vi "Sweep control.vi"(0 "Scan control":cluster{"Priority":u16, "Scan name":u16}[](array[cluster])=[{"Priority"=0, "Scan name"=1}, {"Priority"=3, "Scan name"=0}, {"Priority"=2, "Scan name"=0}, {"Priority"=1, "Scan name"=5}] {"Scan name" items=["OFF", "Vsg1", "Vsg2", "Vsgw", "Vbg", "Field", "Temp"]; "Priority" items=["Priority 0", "Priority 1", "Priority 2", "Priority 3", "Priority 4", "Priority 5"]}, 1 "Scan parameters":T2(array[cluster])=[{"DAQ Channel"=1, "Label"="\nappliedVsg=", "Scaled low"=-0.1, "Scaled high"=0.1, "Start"=0.0, "End"=0.18, "Step"=0.0001, "Scale?"=FALSE}, {"DAQ Channel"=2, "Label"="\nappliedTemperature=", "Scaled low"=-0.175, "Scaled high"=0.775, "Start"=0.1, "End"=0.9, "Step"=0.1, "Scale?"=FALSE}, {"DAQ Channel"=3, "Label"="\nappliedVbg=", "Scaled low"=-0.11, "Scaled high"=0.31, "Start"=-0.5, "End"=0.5, "Step"=0.001, "Scale?"=FALSE}, {"DAQ Channel"=3, "Label"="\nappliedField=", "Scaled low"=-0.060000000000000005, "Scaled high"=0.14, "Start"=-10000.0, "End"=0.0, "Step"=2000.0, "Scale?"=FALSE}] {"Step" format="%#_6f"; "End" format="%#_6f"; "Start" format="%#_6f"; "Scaled high" format="%#_6p"; "Scaled low" format="%#_6p"}, 2 "OSC Configuration":T1(array[cluster])=[{"Signal Type"=enum."Sawtooth Wave", "DC"=0.00034, "Amplitude"=0.0015, "frequency"=0.4, "Phase"=180.0}, {"Signal Type"=enum."Sine Wave", "DC"=0.0, "Amplitude"=0.0, "frequency"=1.0, "Phase"=0.0}, {"Signal Type"=enum."Sine Wave", "DC"=0.0, "Amplitude"=0.0, "frequency"=1.0, "Phase"=0.0}, {"Signal Type"=enum."Sine Wave", "DC"=0.0, "Amplitude"=0.0, "frequency"=1.0, "Phase"=0.0}] {"frequency" format="%0.2p"; "Amplitude" format="%0.2p"; "DC" format="%.2p"}, 3 "Comments":string="SA02704G.20140716\nbackgate=0V", 4 "Experiment folder name":string="3- sweep Vsg_50mK_field", 8 "Additional action (indexing priority)":u16[](array[ring])=[4, 2, 4, 4] items=["Clear DAQ Tasks", "Check Temperature", "Check Field Value", "Wait", "Do Nothing"]) -> ()   [LabVIEW 2013]
uses:
  <userlib>/LevyLab/PPMS_VIs/Lockin-4461_MultiChannel - IV 3.0 globals.vi
panel:
  in  "Number of IV curves":i32=1
  # "Instructions: \n1, you can put multiple scan names in one priority.\n2 OFF has to put in last priority"
  # "I wanted to check the temperature as well as the field (so the zero-field data isn't taken at higher temperatures) so I changed the post-action subvi slightly. In the 'check temperature' case, I made the stop condition that the temp is less than 70mK. By putting 'check temperature' with priority 1, i figure it'll set Vsg1&2 at 0, then wait for the temp to reach 70mK, before it starts sweeping prioity 0."
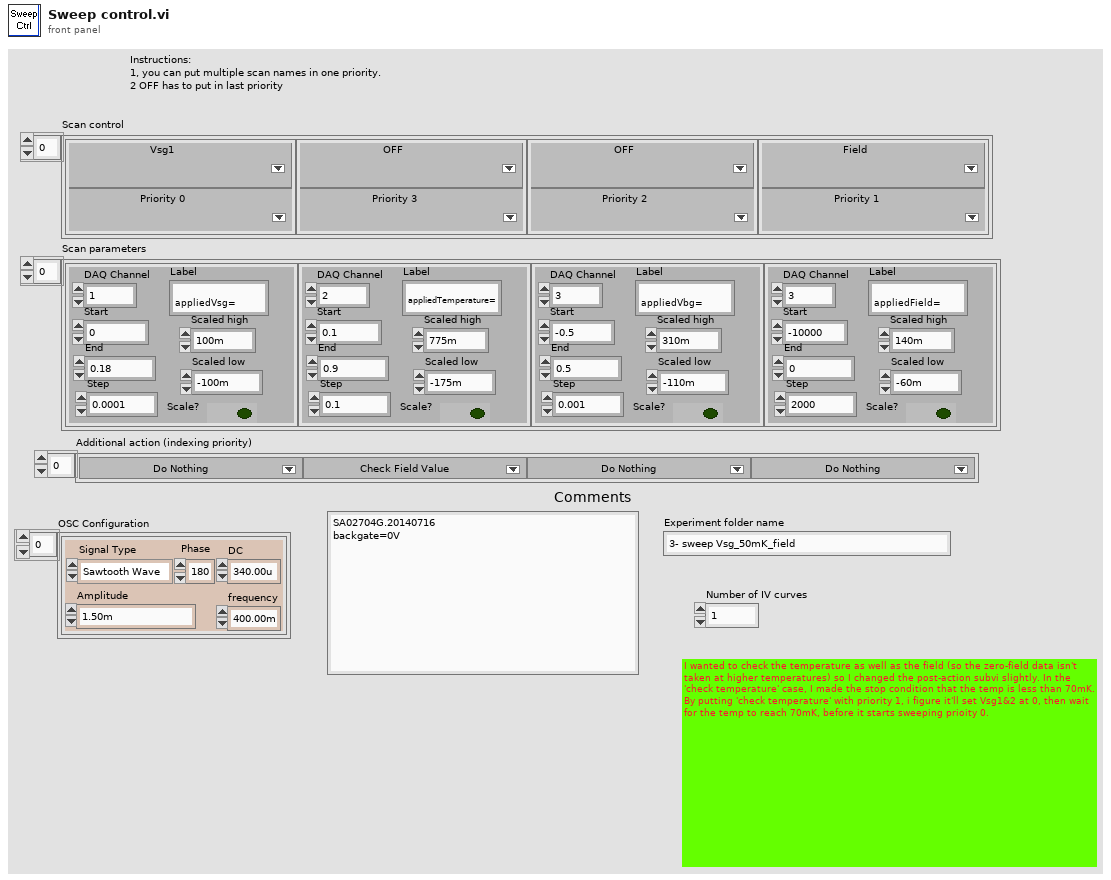
[diagram p1: front panel]
types:
  T1 = cluster{"Signal Type":enum16{"Sine Wave", "Triangle Wave", "Square Wave", "Sawtooth Wave"}, "DC":dbl, "Amplitude":dbl, "frequency":dbl, "Phase":dbl}[]
  T2 = cluster{"DAQ Channel":i32, "Label":string, "Scaled low":dbl, "Scaled high":dbl, "Start":dbl, "End":dbl, "Step":dbl, "Scale?":bool}[]
  T3 = cluster{cluster{"DAQ Channel":i32, "Label":string, "Scaled low":dbl, "Scaled high":dbl, "Start":dbl, "End":dbl, "Step":dbl, "Scale?":bool}[]}[]
  T4 = cluster{cluster{"Priority":u16, "Scan name":u16}[]}[]
  T5 = cluster{cluster{"DAQ Channel":i32, "Label":string, "Scaled low":dbl, "Scaled high":dbl, "Start":dbl, "End":dbl, "Step":dbl, "Scale?":bool}[]}
  T6 = cluster{cluster{"Priority":u16, "Scan name":u16}[]}
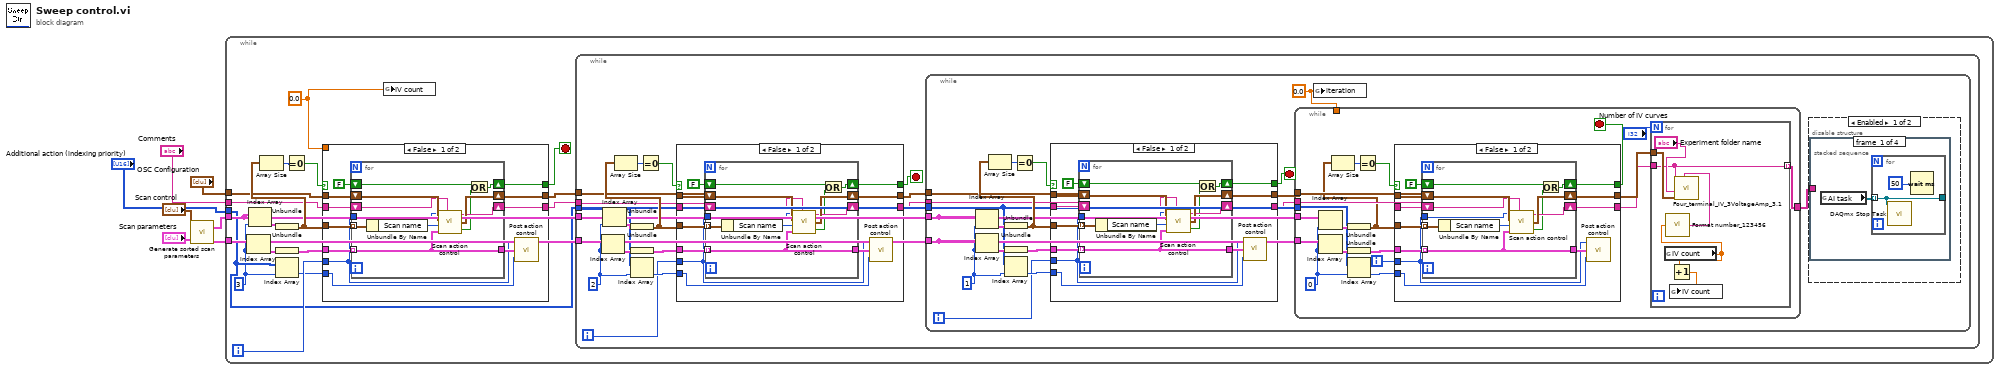
[diagram p0: block diagram]
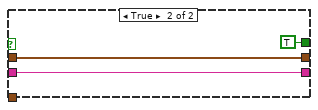
[diagram p2: hidden frame]
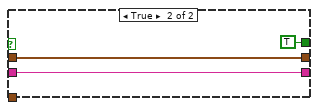
[diagram p3: hidden frame]
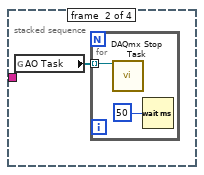
[diagram p4: hidden frame]
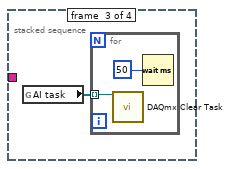
[diagram p5: hidden frame]
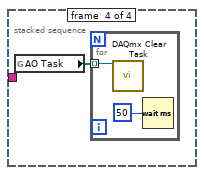
[diagram p6: hidden frame]
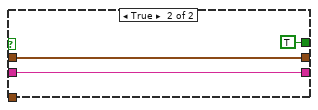
[diagram p8: hidden frame]
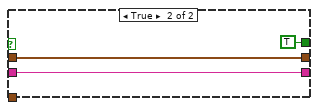
[diagram p9: hidden frame]
diagram:
  n1 = call "Generate sorted scan parameters.vi"("Scan parameters"="Scan parameters", "Scan control"="Scan control") -> ("Sorted scan parameters"=w3:T3, "Sorted scan control"=w2:T4)
  n2 = while {
    tunnel: "Comments" -> [w12]
    tunnel: "OSC Configuration" -> [w13]
    tunnel: w3 -> [w20]
    tunnel: w2 -> [w19]
    tunnel: "Additional action (indexing priority)" -> [w14]
    i -> [w16]
    stop <- w17 stop-if-true
    w8 = 0.0 ("IV count")
    w9 = 3
    n3 = Index Array(array=w20, index=w9) -> (element=w21:T5)
    n4 = Index Array(array=w19, index=w9) -> (element=w18:T6)
    n5 = Unbundle(w18) -> (w23:cluster{"Priority":u16, "Scan name":u16}[])
    n6 = Array Size(array=w23) -> (size(s)=w24:i32)
    n7 = Unbundle(w21) -> (w22:T2)
    n8 = Index Array(array=w14, index=w9) -> (element=w15:u16)
    n9 = Equal To 0?(x=w24) -> (x = 0?=w25:bool)
    n10 = case shown="False" w25 {
      tunnel: w22 -> [w36 _]
      tunnel: [w35 w49] -> w11
      tunnel: [w34 w48] -> w10
      tunnel: [w28 TRUE ("Stop?")] -> w17
      tunnel: w23 -> [w33 _]
      tunnel: w16 -> [w30 _]
      tunnel: w15 -> [w31 _]
      tunnel: w13 -> [w27 w49]
      tunnel: w12 -> [w26 w48]
      tunnel: w8 -> [_ _]
      frame False {
        n11 = for {
          tunnel: w33 -> [w47] mode=indexing
          tunnel: w36 -> [w40] mode=indexing
          tunnel: w30 -> [w41]
          shift-right: [w45] -> w35
          shift-left: w27 -> [w44]
          shift-right: [w43] -> w34
          shift-left: w26 -> [w42]
          tunnel: [w40] -> w32
          shift-right: [w37] -> w28
          shift-left: FALSE -> [w39]
          n12 = Unbundle By Name(w47) -> ("Scan name"=w46:u16)
          n13 = call "Scan action control.vi"("Index"=w41, "OSC Configuration"=w44, "Scan control"=w46, "Scan Parameters"=w40, "Comments"=w42) -> ("Comments out"=w43:string, "OSC Configuration out"=w45:T1, "Stop?"=w38:bool)
          n14 = Or(x=w39, y=w38) -> (x .or. y?=w37:bool)
        }
        n15 = call "Post action control.vi"("Action"=w31, "Scan Parameters"=w32, "Index"=w30) -> ()  [unwired: 1 out]
      }
      frame True {
      }
    }
    n16 = global write "Lockin-4461_MultiChannel - IV 3.0 globals.vi" "IV count"(w8) -> ()
    n17 = while {
      tunnel: w20 -> [w60]
      tunnel: w19 -> [w59]
      tunnel: w14 -> [w58]
      tunnel: w10 -> [w57]
      tunnel: w11 -> [w56]
      i -> [w55]
      stop <- w54 stop-if-true
      w51 = 2
      n18 = Index Array(array=w60, index=w51) -> (element=w66:T5)
      n19 = Index Array(array=w59, index=w51) -> (element=w67:T6)
      n20 = Unbundle(w67) -> (w64:cluster{"Priority":u16, "Scan name":u16}[])
      n21 = Array Size(array=w64) -> (size(s)=w62:i32)
      n22 = Unbundle(w66) -> (w65:T2)
      n23 = Index Array(array=w58, index=w51) -> (element=w63:u16)
      n24 = Equal To 0?(x=w62) -> (x = 0?=w61:bool)
      n25 = case shown="False" w61 {
        tunnel: w65 -> [w78 _]
        tunnel: w56 -> [w77 w92]
        tunnel: w57 -> [w76 w91]
        tunnel: [w75 w92] -> w53
        tunnel: [w74 w91] -> w52
        tunnel: [w68 TRUE ("Stop?")] -> w54
        tunnel: w64 -> [w73 _]
        tunnel: w55 -> [w70 _]
        tunnel: w63 -> [w71 _]
        frame False {
          n26 = for {
            tunnel: w73 -> [w89] mode=indexing
            tunnel: w78 -> [w82] mode=indexing
            tunnel: w70 -> [w83]
            shift-right: [w87] -> w75
            shift-left: w77 -> [w86]
            shift-right: [w85] -> w74
            shift-left: w76 -> [w84]
            tunnel: [w82] -> w72
            shift-right: [w79] -> w68
            shift-left: FALSE -> [w81]
            n27 = Unbundle By Name(w89) -> ("Scan name"=w88:u16)
            n28 = call "Scan action control.vi"("Index"=w83, "OSC Configuration"=w86, "Scan control"=w88, "Scan Parameters"=w82, "Comments"=w84) -> ("Comments out"=w85:string, "OSC Configuration out"=w87:T1, "Stop?"=w80:bool)
            n29 = Or(x=w81, y=w80) -> (x .or. y?=w79:bool)
          }
          n30 = call "Post action control.vi"("Action"=w71, "Scan Parameters"=w72, "Index"=w70) -> ()  [unwired: 1 out]
        }
        frame True {
        }
      }
      n31 = while {
        tunnel: w53 -> [w102]
        tunnel: w52 -> [w101]
        tunnel: w59 -> [w100]
        tunnel: w60 -> [w99]
        tunnel: w58 -> [w98]
        i -> [w93]
        stop <- w95 stop-if-true
        w94 = 1
        w111 = 0.0 ("iteration")
        n32 = Index Array(array=w100, index=w94) -> (element=w103:T6)
        n33 = Index Array(array=w99, index=w94) -> (element=w104:T5)
        n34 = Unbundle(w103) -> (w106:cluster{"Priority":u16, "Scan name":u16}[])
        n35 = Array Size(array=w106) -> (size(s)=w108:i32)
        n36 = Unbundle(w104) -> (w105:T2)
        n37 = Index Array(array=w98, index=w94) -> (element=w107:u16)
        n38 = Equal To 0?(x=w108) -> (x = 0?=w109:bool)
        n39 = case shown="False" w109 {
          tunnel: w105 -> [w135 _]
          tunnel: w102 -> [w134 w149]
          tunnel: w101 -> [w133 w148]
          tunnel: [w132 w149] -> w96
          tunnel: [w131 w148] -> w97
          tunnel: [w125 TRUE ("Stop?")] -> w95
          tunnel: w106 -> [w130 _]
          tunnel: w93 -> [w127 _]
          tunnel: w107 -> [w128 _]
          frame False {
            n40 = for {
              tunnel: w130 -> [w146] mode=indexing
              tunnel: w135 -> [w139] mode=indexing
              tunnel: w127 -> [w140]
              shift-right: [w144] -> w132
              shift-left: w134 -> [w143]
              shift-right: [w142] -> w131
              shift-left: w133 -> [w141]
              tunnel: [w139] -> w129
              shift-right: [w136] -> w125
              shift-left: FALSE -> [w138]
              n41 = Unbundle By Name(w146) -> ("Scan name"=w145:u16)
              n42 = call "Scan action control.vi"("Index"=w140, "OSC Configuration"=w143, "Scan control"=w145, "Scan Parameters"=w139, "Comments"=w141) -> ("Comments out"=w142:string, "OSC Configuration out"=w144:T1, "Stop?"=w137:bool)
              n43 = Or(x=w138, y=w137) -> (x .or. y?=w136:bool)
            }
            n44 = call "Post action control.vi"("Action"=w128, "Scan Parameters"=w129, "Index"=w127) -> ()  [unwired: 1 out]
          }
          frame True {
          }
        }
        n45 = while {
          tunnel: w100 -> [w167]
          tunnel: w99 -> [w166]
          tunnel: w96 -> [w162]
          tunnel: w97 -> [w161]
          tunnel: w98 -> [w155]
          tunnel: w111 -> [_]
          tunnel: [w151] -> w110
          i -> [w156]
          stop <- w158 stop-if-true
          w150 = 0
          n46 = Index Array(array=w167, index=w150) -> (element=w165:T6)
          n47 = Index Array(array=w166, index=w150) -> (element=w164:T5)
          n48 = Unbundle(w165) -> (w157:cluster{"Priority":u16, "Scan name":u16}[])
          n49 = Array Size(array=w157) -> (size(s)=w153:i32)
          n50 = Unbundle(w164) -> (w163:T2)
          n51 = Index Array(array=w155, index=w150) -> (element=w154:u16)
          n52 = Equal To 0?(x=w153) -> (x = 0?=w152:bool)
          n53 = case shown="False" w152 {
            tunnel: w163 -> [w179 _]
            tunnel: w162 -> [w178 w193]
            tunnel: w161 -> [w177 w192]
            tunnel: [w176 w193] -> w160
            tunnel: [w175 w192] -> w159
            tunnel: [w169 TRUE ("Stop?")] -> w158
            tunnel: w157 -> [w174 _]
            tunnel: w156 -> [w171 _]
            tunnel: w154 -> [w172 _]
            frame False {
              n54 = for {
                tunnel: w174 -> [w190] mode=indexing
                tunnel: w179 -> [w183] mode=indexing
                tunnel: w171 -> [w184]
                shift-right: [w188] -> w176
                shift-left: w178 -> [w187]
                shift-right: [w186] -> w175
                shift-left: w177 -> [w185]
                tunnel: [w183] -> w173
                shift-right: [w180] -> w169
                shift-left: FALSE -> [w182]
                n55 = Unbundle By Name(w190) -> ("Scan name"=w189:u16)
                n56 = call "Scan action control.vi"("Index"=w184, "OSC Configuration"=w187, "Scan control"=w189, "Scan Parameters"=w183, "Comments"=w185) -> ("Comments out"=w186:string, "OSC Configuration out"=w188:T1, "Stop?"=w181:bool)
                n57 = Or(x=w182, y=w181) -> (x .or. y?=w180:bool)
              }
              n58 = call "Post action control.vi"("Action"=w172, "Scan Parameters"=w173, "Index"=w171) -> ()  [unwired: 1 out]
            }
            frame True {
            }
          }
          n59 = for {
            N: "Number of IV curves" -> [_]
            tunnel: w160 -> [w196]
            tunnel: w159 -> [w195]
            tunnel: [w195] -> w151 mode=indexing
            n60 = global read "Lockin-4461_MultiChannel - IV 3.0 globals.vi" "IV count"() -> (w198:dbl)
            n61 = call <userlib>:"Format number_123456.vi"("number"=w198) -> ("String"=w194:string)
            n62 = Increment(x=w198) -> (x+1=w199:dbl)
            n63 = global write "Lockin-4461_MultiChannel - IV 3.0 globals.vi" "IV count"(w199) -> ()
            n64 = call <userlib>:"Four_terminal_IV_3VoltageAmp_3.1.vi"("Initial index (000000)"=w194, "OSC Configuration"=w196, "Experiment folder name"="Experiment folder name", "Comments"=w195) -> ()  [unwired: 1 in, 5 out]
          }
        }
        n65 = global write "Lockin-4461_MultiChannel - IV 3.0 globals.vi" "iteration"(w111) -> ()
        n66 = disable-structure shown="Enabled" {
          disable-tunnel: w110 -> [w112 _]
          frame Enabled {
            n67 = stacked-sequence {
              tunnel: w112 -> [_ _ _ _]
              frame #0 {
                n68 = global read "Lockin-4461_MultiChannel - IV 3.0 globals.vi" "AI task"() -> (w113:refnum<k21>[])
                n69 = for {
                  tunnel: w113 -> [w114] mode=indexing
                  tunnel: [w114] -> _
                  n70 = call <vilib>:"DAQmx Stop Task.vi"("task/channels in"=w114) -> ()  [unwired: 13 in, 2 out]
                  n71 = Wait (ms)(milliseconds to wait=u32 50) -> ()  [unwired: 1 out]
                }
              }
              frame #1 {
                n72 = global read "Lockin-4461_MultiChannel - IV 3.0 globals.vi" "AO Task"() -> (w116:refnum<k21>[])
                n73 = for {
                  tunnel: w116 -> [w118] mode=indexing
                  n74 = call <vilib>:"DAQmx Stop Task.vi"("task/channels in"=w118) -> ()  [unwired: 13 in, 2 out]
                  n75 = Wait (ms)(milliseconds to wait=u32 50) -> ()  [unwired: 1 out]
                }
              }
              frame #2 {
                n76 = global read "Lockin-4461_MultiChannel - IV 3.0 globals.vi" "AI task"() -> (w119:refnum<k21>[])
                n77 = for {
                  tunnel: w119 -> [w121] mode=indexing
                  n78 = call <vilib>:"DAQmx Clear Task.vi"("task in"=w121) -> ()  [unwired: 14 in, 1 out]
                  n79 = Wait (ms)(milliseconds to wait=u32 50) -> ()  [unwired: 1 out]
                }
              }
              frame #3 {
                n80 = global read "Lockin-4461_MultiChannel - IV 3.0 globals.vi" "AO Task"() -> (w122:refnum<k21>[])
                n81 = for {
                  tunnel: w122 -> [w124] mode=indexing
                  n82 = call <vilib>:"DAQmx Clear Task.vi"("task in"=w124) -> ()  [unwired: 14 in, 1 out]
                  n83 = Wait (ms)(milliseconds to wait=u32 50) -> ()  [unwired: 1 out]
                }
              }
            }
          }
          frame Disabled {
          }
        }
      }
    }
  }
